vi "ziGetEventByteArray.vi"(8 "Error In":errorcluster, 10 "ByteArray In":T1={"Timestamp (ticks)"=2149, "bytes"=[]}, 11 "Handle In":T2 {"Handle" format="0x%08x"; "Conn" format="0x%08x"}) -> (0 "Error Out":errorcluster, 2 "ByteArray Out":T1={"Timestamp (ticks)"=2149, "bytes"=[]}, 3 "Handle Out":T2 {"Handle" format="0x%08x"; "Conn" format="0x%08x"})   [LabVIEW 2015, in "Zurich Instruments LabOne.lvlib"]
uses:
  Zurich Instruments LabOne.lvlib
  Zurich Instruments/LabOne/API/LabVIEW/Zurich Instruments LabOne/Private/ziLV64.framework
  ziTypeHandle.ctl
  ziTypeByteArray.ctl
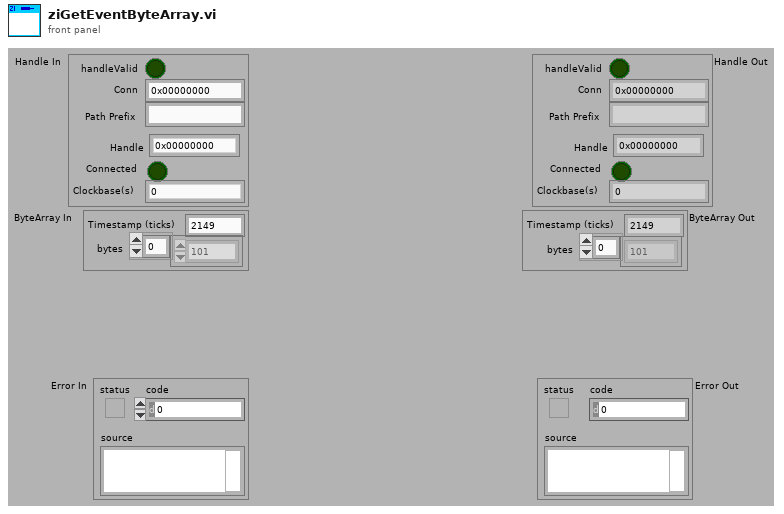
[diagram p1: front panel]
types:
  T1 = typedef "Zurich Instruments LabOne.lvlib/ziTypeByteArray.ctl" = cluster{"Timestamp (ticks)":u64, "bytes":i8[]}
  T2 = typedef "Zurich Instruments LabOne.lvlib/ziTypeHandle.ctl" = cluster{"handleValid":bool, "Conn":u64, "Path Prefix":string, "Handle":u64, "Connected":bool, "Clockbase(s)":dbl}
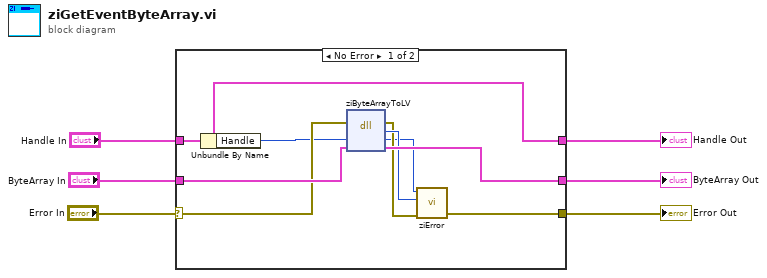
[diagram p0: block diagram]
diagram:
  n1 = case shown="No Error" "Error In" {
    selector: "Error In" -> [w12 w18]
    tunnel: "Handle In" -> [w8 w16]
    tunnel: [w8 w16] -> w5
    tunnel: [w15 w17] -> w4
    tunnel: "ByteArray In" -> [w14 w17]
    tunnel: [w13 w18] -> w2
    frame No Error {
      n2 = Unbundle By Name(w8) -> ("Handle"=w10:u64)
      n3 = dll-call lib="Users/arkady/Desktop/ado/github/resonant_ultrasound_arxiv/maglab ultrasound -- arkady --arxiv/Zurich Instruments/LabOne/API/LabVIEW/Zurich Instruments LabOne/Private/ziLV*.*" fn="ziByteArrayToLV"(error in=w12, "ziEventBuffer"=w10, "byteArray"=w14) -> (error out=w9:errorcluster, "return type"=w11:u32, "ziEventBuffer"=w7:u64, "byteArray"=w15:T1)  [unwired: 2 in, 1 out]
      n4 = call "ziError.vi"("Conn"=w7, "ziErrorCode"=w11, "Error In"=w9) -> ("Error Out"=w13:errorcluster)  [unwired: 2 in, 1 out]
    }
    frame Error {
    }
  }
  "Handle Out" <- w5
  "ByteArray Out" <- w4
  "Error Out" <- w2
